vi "Check Context Dependent Rings.vi"(0 "Display State in":T1, 11 "ItemNames in":string[][](array[string]), 13 "CellPosition":T6) -> (4 "Display State out":T1, 15 "ItemNames out":string[][](array[string]))   [LabVIEW 2015, in "KTable.xctl"]
uses:
  KTable.xctl
  <vilib>/Utility/miscctls.llb/LVRowAndColumnTypeDef.ctl
  State.ctl
  ColumnSpec.ctl
  ColumnType.ctl
  Table Properties.ctl
  Events.ctl
  Event Data.ctl
  Event Type.ctl
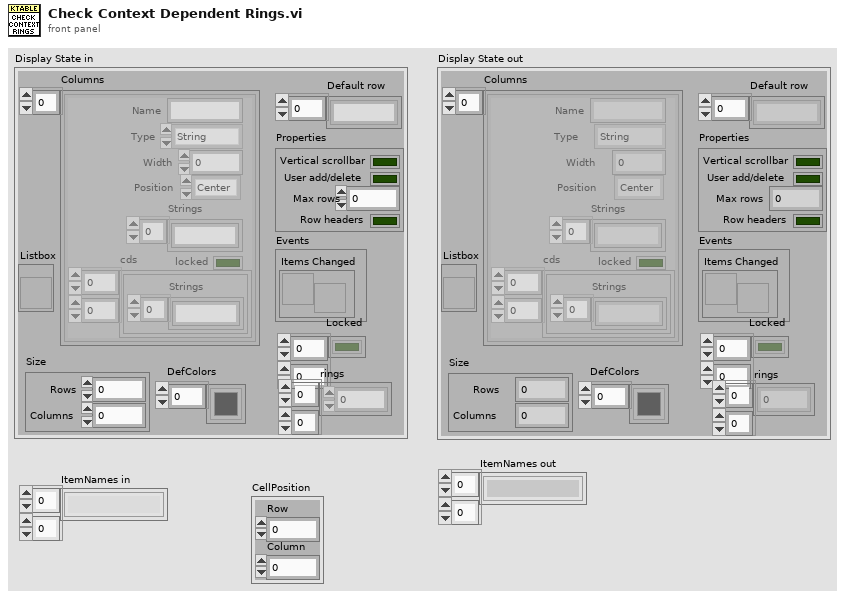
[diagram p1: front panel]
types:
  T1 = typedef "KTable.xctl/State.ctl" = cluster{"Columns":T2[], "Listbox":refnum<vi>, "Default row":string[], "Properties":T4, "Events":T5, "Locked":bool[][], "Size":cluster{"Rows":i32, "Columns":i32}, "rings":i32[][], "DefColors":u32[]}
  T2 = typedef "KTable.xctl/ColumnSpec.ctl" = cluster{"Name":string, "Type":T3, "Width":i32, "Strings":string[], "Position":enum16{"Left", "Center", "Right"}, "locked":bool, "cds":cluster{"Strings":string[]}[][]}
  T3 = typedef "KTable.xctl/ColumnType.ctl" = enum16{"String", "Enum", "Int", "Double", "Boolean", "Ring", "Formula", "Color"}
  T4 = typedef "KTable.xctl/Table Properties.ctl" = cluster{"Vertical scrollbar":bool, "User add/delete":bool, "Max rows":i32, "Row headers":bool}
  T5 = typedef "KTable.xctl/Events.ctl" = cluster{"Items Changed":refnum<user-event>}
  T6 = typedef "LVRowAndColumnTypeDef.ctl" = cluster{"Row":i32, "Column":i32}
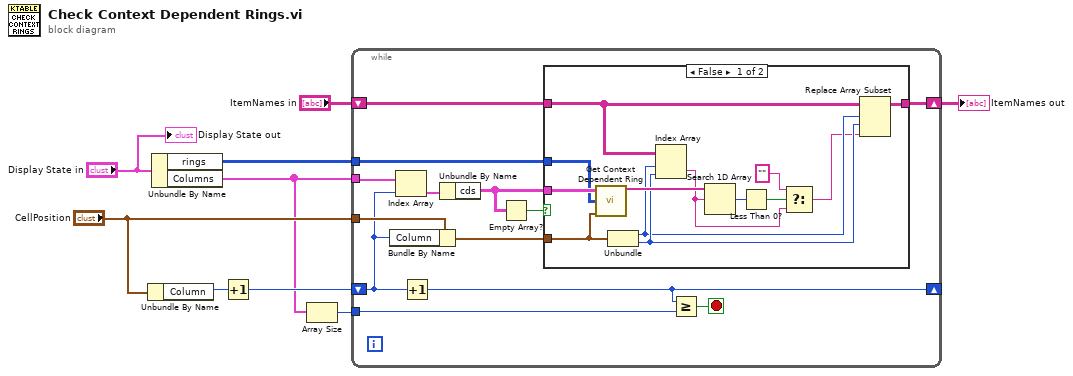
[diagram p0: block diagram]
diagram:
  n1 = Unbundle By Name("CellPosition") -> ("Column"=w9:i32)
  n2 = Unbundle By Name("Display State in") -> ("rings"=w6:i32[][], "Columns"=w5:T2[])
  n3 = Increment(x=w9) -> (x+1=w8:i32)
  n4 = Array Size(array=w5) -> (size(s)=w4:i32)
  n5 = while {
    shift-right: [w14] -> _
    shift-left: w8 -> [w15]
    tunnel: w5 -> [w22]
    tunnel: "CellPosition" -> [w20]
    tunnel: w6 -> [w17]
    tunnel: w4 -> [w13]
    shift-right: [w10] -> w1
    shift-left: "ItemNames in" -> [w11]
    stop <- w12 stop-if-true
    n6 = Bundle By Name(cluster=w20, "Column"=w15) -> (w16:T6)
    n7 = Index Array(array=w22, index=w15) -> (element=w21:T2)
    n8 = Increment(x=w15) -> (x+1=w14:i32)
    n9 = Unbundle By Name(w21) -> ("cds"=w19:cluster{"Strings":string[]}[][])
    n10 = Empty Array?(array=w19) -> (empty?=w18:bool)
    n11 = case shown="False" w18 {
      tunnel: w19 -> [w35 _]
      tunnel: w17 -> [w34 _]
      tunnel: w16 -> [w33 _]
      tunnel: w11 -> [w30 w36]
      tunnel: [w29 w36] -> w10
      frame False {
        n12 = call "Get Context Dependent Ring.vi"("cds"=w35, "rings"=w34, "Cell Position"=w33) -> ("Strings"=w32:string[])  [unwired: 12 in]
        n13 = Unbundle(w33) -> ("Row"=w27:i32, "Column"=w28:i32)
        n14 = Index Array(array=w30, index (row)=w27, index (col)=w28) -> (element=w23:string)
        n15 = Search 1D Array(1D array=w32, element=w23) -> (index of element=w31:i32)  [unwired: 1 in]
        n16 = Less Than 0?(x=w31) -> (x < 0?=w26:bool)
        n17 = Select(t="", s=w26, f=w23) -> (s? t:f=w24:string)
        n18 = Replace Array Subset(array=w30, new element=w24, index (row)=w27, index (col)=w28) -> (w29:string[][])
      }
      frame True {
      }
    }
    n19 = Greater Or Equal?(x=w14, y=w13) -> (x >= y?=w12:bool)
  }
  "ItemNames out" <- w1
  "Display State out" <- "Display State in"
